vi "Calculate S.vi"(0 "Chi_CO2_A":dbl format="%#_13g", 1 "Chi_CO2_B":dbl format="%#_13g", 2 "Chi_H2O_A":dbl format="%#_13g", 3 "Chi_H2O_B":dbl format="%#_13g", 4 "Raw_CO2_A":dbl format="%#_13g", 5 "Raw_CO2_B":dbl format="%#_13g", 8 "Z":dbl format="%#_13g", 9 "T [C]":dbl format="%#_13g", 11 "P [hpa]":dbl format="%#_13g") -> (16 "S":dbl)   [LabVIEW 2010]
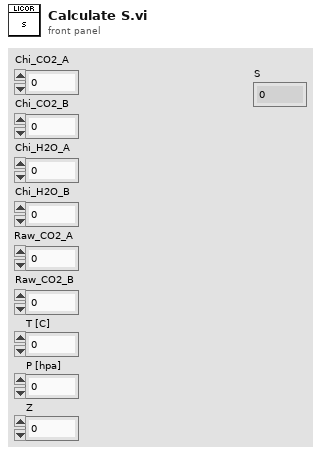
[diagram p1: front panel]
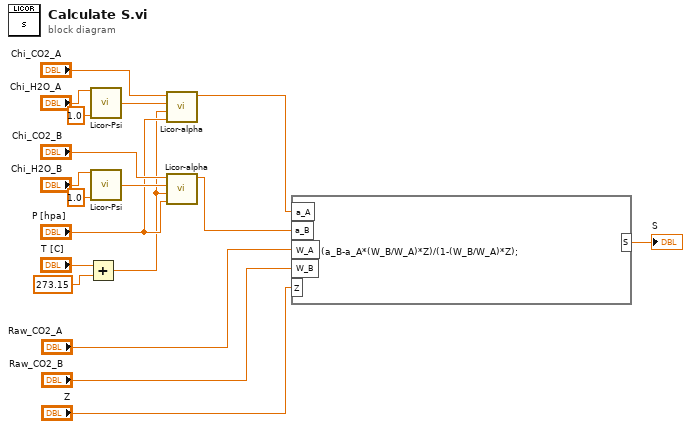
[diagram p0: block diagram]
diagram:
  n1 = Add(x="T [C]", y=273.15) -> (x+y=w12:dbl)
  n2 = call "Licor-Psi.vi"("Chi_i"="Chi_H2O_A", "a"=1.0) -> ("Psi_i"=w14:dbl)  [unwired: 13 in]
  n3 = call "Licor-Psi.vi"("Chi_i"="Chi_H2O_B", "a"=1.0) -> ("Psi_i"=w15:dbl)  [unwired: 13 in]
  n4 = call "Licor-alpha.vi"("P [kPa]"="P [hpa]", "T [K]"=w12, "Psi_i"=w14, "Chi_i"="Chi_CO2_A") -> ("absorptance_i"=w9:dbl)  [unwired: 7 in]
  n5 = call "Licor-alpha.vi"("P [kPa]"="P [hpa]", "T [K]"=w12, "Psi_i"=w15, "Chi_i"="Chi_CO2_B") -> ("absorptance_i"=w10:dbl)  [unwired: 7 in]
  n6 = formula code="S = (a_B-a_A*(W_B/W_A)*Z)/(1-(W_B/W_A)*Z);"("a_B"=w10, "a_A"=w9, "W_A"="Raw_CO2_A", "W_B"="Raw_CO2_B", "Z"="Z") -> ("S"=→"S":dbl)
